vi "On Start.vi"(8 "error in":errorcluster, 9 "Channel Settings":T1[](array[typedef]), 10 "Append data?":bool, 11 "file path":path) -> (0 "error out":errorcluster, 3 "file reference":refnum<file>)   [LabVIEW 2021, in "Logging.lvlib"]
doc: "Open the data log file in 'file path'. If 'Append data?' is FALSE, create an empty file and write a header with columns for timestamps and channel names according to 'Channel Settings'. If 'Append data?' is TRUE, open the data log file and seek to its end."
uses:
  Logging.lvlib
  Acquisition/Channel Settings.ctl
  Acquisition/IO Device.ctl
  Acquisition/Acquisition.lvlib
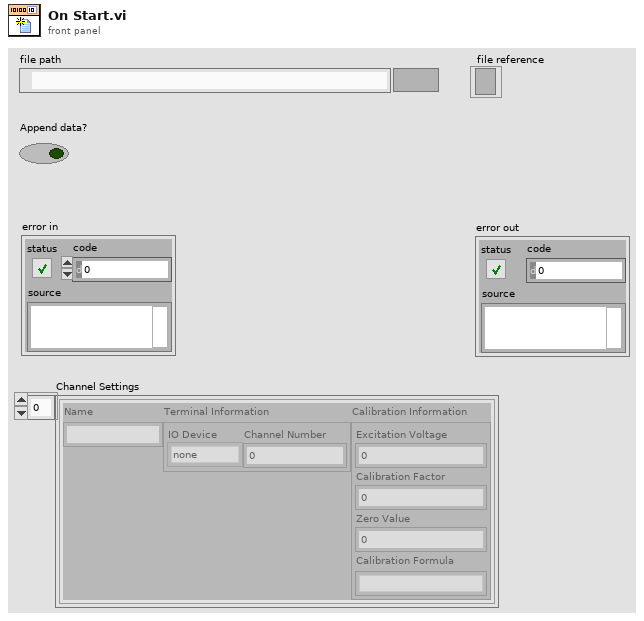
[diagram p1: front panel]
types:
  T1 = typedef "Acquisition.lvlib/Channel Settings.ctl" = cluster{"Name":string, "Terminal Information":cluster{"IO Device":T2, "Channel Number":i32}, "Calibration Information":cluster{"Excitation Voltage":dbl, "Calibration Factor":dbl, "Zero Value":dbl, "Calibration Formula":string}}
  T2 = typedef "Acquisition.lvlib/IO Device.ctl" = enum16{"none", "9219", "9401"}
  T3 = enum16{"open", "replace", "create", "open or create", "replace or create", "replace or create with confirmation"}
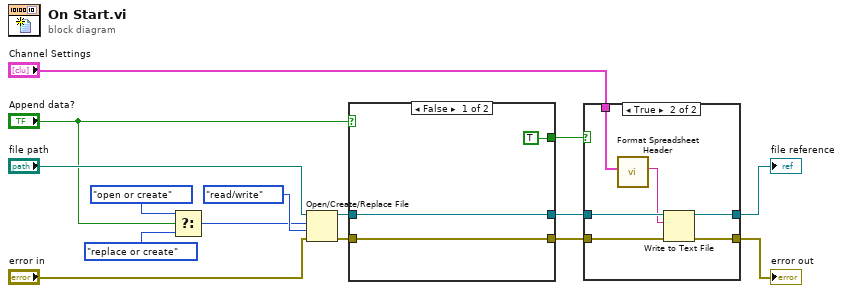
[diagram p0: block diagram]
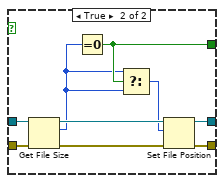
[diagram p3: hidden frame]
diagram:
  n1 = Select(t=T3."open or create" ("operation (0:open)"), s="Append data?", f=T3."replace or create" ("operation (0:open)")) -> (s? t:f=w9:T3)
  n2 = Open/Create/Replace File(file path (use dialog)="file path", error in="error in", operation (0:open)=w9, access (0:read/write)=enum16{"read/write", "read-only", "write-only"}."read/write") -> (refnum out=w6:refnum<file>, error out=w5:errorcluster)  [unwired: 2 in, 1 out]
  n3 = case shown="False" "Append data?" {
    tunnel: w6 -> [w17 w26]
    tunnel: w5 -> [w18 w25]
    tunnel: [w18 w23] -> w2
    tunnel: [w17 w22] -> w3
    tunnel: [TRUE w21] -> w4
    frame False {
    }
    frame True {
      n4 = Get File Size(file=w26, error in=w25) -> (refnum out=w27:refnum<file>, size (in bytes)=w19:i64, 0:w24:errorcluster)
      n5 = Equal To 0?(x=w19) -> (x = 0?=w21:bool)
      n6 = Select(t=w19, s=w21, f=w19) -> (s? t:f=w20:i64)
      n7 = Set File Position(offset (in bytes) (0)=w20, refnum=w27, error in=w24) -> (refnum out=w22:refnum<file>, error out=w23:errorcluster)  [unwired: 1 in]
    }
  }
  n8 = case shown="True" w4 {
    tunnel: [w28 w35] -> w12
    tunnel: [w29 w34] -> w11
    tunnel: w3 -> [w29 w33]
    tunnel: w2 -> [w28 w32]
    tunnel: "Channel Settings" -> [_ w30]
    frame False {
    }
    frame True {
      n9 = call "Format Spreadsheet Header.vi"("Channel Settings"=w30) -> ("Log file header"=w31:string)  [unwired: 10 in]
      n10 = Write to Text File(file (use dialog)=w33, text=w31, error in=w32) -> (refnum out=w34:refnum<file>, error out=w35:errorcluster)  [unwired: 1 in, 1 out]
    }
  }
  "file reference" <- w11
  "error out" <- w12
